vi "Arm Aircraft.vi"(8 "Error In":errorcluster, 11 "ARM(T)/DISARM(F)":bool=TRUE) -> (0 "error out":errorcluster, 3 "Selected Aircraft ID Out":u8)   [LabVIEW 2014]
uses:
  Aircraft Information/Sub VI/Selected Aircraft/SubVI/Get Selected Aircraft.vi
  Commands/MAV_CMD Sub VI/MAV_CMD_COMPONENT_ARM_DISARM.vi
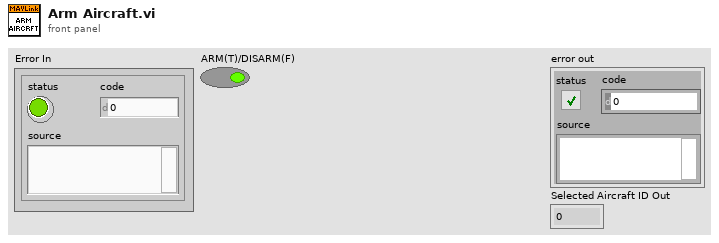
[diagram p1: front panel]
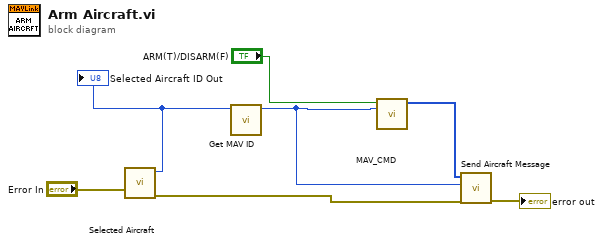
[diagram p0: block diagram]
diagram:
  n1 = call-poly "Selected Aircraft.vi"("Error In"="Error In") -> ("Error Out"=w5:errorcluster, "Selected Aircraft ID Out"=w6:u8)  [unwired: 9 in]
  "Selected Aircraft ID Out" <- w6
  n2 = call "Get MAV ID.vi"("Aircraft Index"=w6) -> ("Aircraft ID"=w4:u8)  [unwired: 9 in, 1 out]
  n3 = call-poly "MAV_CMD.vi"("Target System and Target Component"=w4, "ARM(T)/DISARM(F)"="ARM(T)/DISARM(F)") -> ("MAVLink Message"=w7:u8[])  [unwired: 9 in]
  n4 = call "Send Aircraft Message.vi"("error in (no error)"=w5, "Aircraft ID"=w4, "MAVLink Message"=w7) -> ("error out"=→"error out":errorcluster)  [unwired: 8 in]
